vi "Convert State For Save.vi"(2 "Container State":T1, 3 "Display State":T2) -> (1 "Display State To Save":variant)   [LabVIEW 2017, in "XY Plot Matrix.xctl"]
uses:
  <vilib>/Math Plots/2D Math Plots/XY Plot Matrix/XY Plot Matrix XCtrl/XY Plot Matrix.xctl
  <vilib>/Math Plots/2D Math Plots/XY Plot Matrix/XY Plot Matrix XCtrl/State.ctl
  <vilib>/Math Plots/2D Math Plots/XY Plot Matrix/XY Plot Matrix/XY Plot Matrix.lvclass
  e:/builds/penguin/labview/branches/2017/dev/dist/vi.lib/Math Plots/2D Math Plots/2D Plot/2D Plot/2D Plot.lvclass
  <vilib>/Math Plots/2D Math Plots/2D Plot/Action String/XYPlotMatrix Ctrl Act Queue.ctl
  <vilib>/Math Plots/2D Math Plots/2D Plot/Action String/XYPlotMatrix Ctrl Act Cluster.ctl
  <vilib>/Math Plots/2D Math Plots/2D Plot/Action String/2DMathPlot State Class.ctl
  <vilib>/_xctls/Container State.ctl
  <vilib>/Math Plots/2D Math Plots/2D Plot/2D Plot/2D Plot.lvclass
  <vilib>/_xctls/XControlSupport.lvlib
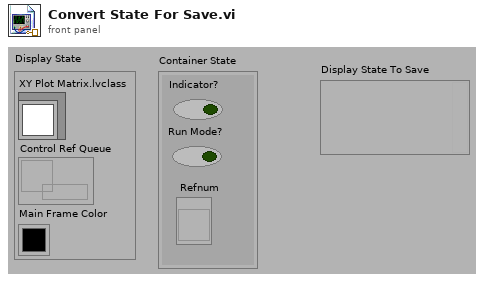
[diagram p1: front panel]
types:
  T1 = typedef "XControlSupport.lvlib/Container State.ctl" = cluster{"Indicator?":bool, "Run Mode?":bool, " Refnum":refnum<vi>}
  T2 = typedef "XY Plot Matrix.xctl/State.ctl" = cluster{"XY Plot Matrix.lvclass":refnum<class "XY Plot Matrix.lvclass">, "Control Ref Queue":T3, "Main Frame Color":u32}
  T3 = typedef "XYPlotMatrix Ctrl Act Queue.ctl" = refnum<queue>
  T4 = typedef "XYPlotMatrix Ctrl Act Cluster.ctl" = cluster{"Facade VI":refnum<vi>, "XControl":refnum<vi>, "Sub Panel":refnum<vi>, "Sub VI":refnum<vi>, "Export Image":refnum<vi>, "Display State Change Class":T5}
  T5 = typedef "2DMathPlot State Class.ctl" = enum16{"Update All (Undo)", "Update General", "Update Appearance", "Update Format", "Update Scale", "Update Marker", "Update Cursor", "None"}
  T6 = typedef "XY Plot Matrix.lvclass/Plotmatrix Property Array Cluster.ctl" = cluster{"Plotmatrix Property Array":T7, "Active Position":T11}
  T7 = typedef "XY Plot Matrix.lvclass/Plotmatrix Property Array.ctl" = T8[][]
  T8 = typedef "XY Plot Matrix.lvclass/Plotmatrix Property.ctl" = cluster{"Plot Property Array":T9}
  T9 = typedef "2D Plot.lvclass/Plot Property Array.ctl" = T10[]
  T10 = typedef "2D Plot.lvclass/Plot Property.ctl" = cluster{"Bar Plot Style":u8, "DigitalLineStyle":u8, "TransitionLocation":u8, "Transition Type":u8, "Fill To":i16, "Fill/Pt. Color":u32, "Label Style":u8, "Line Style":u8, "Line Width":u8, "Plot Color":u32, "Plot Interpolation":u8, "Plot Name":string, "Point Style":u8, "Visible?":bool, "XScaleIdx":u32, "YScaleIdx":u32}
  T11 = typedef "XY Plot Matrix.lvclass/Active Position.ctl" = cluster{"Row":i32, "Column":i32}
  T12 = typedef "2D Plot.lvclass/Property Cluster.ctl" = cluster{"Graph General":T13, "Format Property":string[], "Scale Array":T14, "Cursor Property":T17, "Annotation List":T19, "Active Cursor":i32, "Active Plot":i32}
  T13 = typedef "2D Plot.lvclass/Graph General Property.ctl" = cluster{"Palette Visible":cluster{"Graph Legend":bool, "Plot Legend":bool, "Auto size":bool, "Number of Plots":u32, "X Scrollbar":bool, "Scale Legend":bool, "Cursor Legend":bool}, "Plot Area Color":cluster{"FG Color":u32, "BG Color":u32}, "Bounds Size":cluster{"Width":u32, "Height":u32}, "Plot Area Bounds":cluster{"Left":i16, "Top":i16, "Right":i16, "Bottom":i16}}
  T14 = typedef "2D Plot.lvclass/Scale Array.ctl" = T15[]
  T15 = typedef "2D Plot.lvclass/Scale Cluster.ctl" = cluster{"General":cluster{"Editable":bool, "Flipped":bool, "Mapping Mode":u8, "Visible":bool, "Style":u8, "Scale Fit":u8}, "Offset and Multiplier":T16, "Range":cluster{"Minimum":dbl, "Maximum":dbl, "Increment":dbl, "Minor Increment":dbl, "Start":dbl}, "Tick Color":cluster{"Major Color":u32, "Minor Color":u32}, "Gird Color":cluster{"Major Color":u32, "Minor Color":u32}, "Marker":cluster{"Visible":bool, "FG Color":u32, "BG Color":u32, "Font Name":string, "Font Size":u32, "Font Bold":bool, "Font Italic":bool, "Font Strikeout":bool, "Font Underline":bool}, "Name Label":cluster{"Visible":bool, "FG Color":u32, "BG Color":u32, "Font Name":string, "Font Size":u32, "Font Bold":bool, "Font Italic":bool, "Font Strikeout":bool, "Font Underline":bool, "Justification":enum16{"Left", "Center", "Right"}, "Text":string}}
  T16 = typedef "LVOffsetAndMultiplierTypeDef.ctl" = cluster{"Offset":dbl, "Multiplier":dbl}
  T17 = typedef "2D Plot.lvclass/Cursor Property.ctl" = cluster{"Cursor List":T18, "Cursor List Addtional":cluster{"Cursor Selection Color":u32, "Line Style":u8, "Line Width":u8, "Visible":bool}[]}
  T18 = typedef "LVCursorListTypeDef.ctl" = cluster{"Name":string, "Color":u32, "Style":u8, "Point Style":u8, "Name Visible":bool, "Allow Drag":bool, "Cursor Mode":u32, "Plot":i32, "Index":i32, "Position":cluster{"X":dbl, "Y":dbl}, "X Scale":u32, "Y Scale":u32, "Watch Plots":i32[], "Watch All Plots":bool, "Plot Area":i32, "Label Offset":cluster{"X":dbl, "Y":dbl}}[]
  T19 = typedef "LVAnnotationListTypeDef.ctl" = cluster{"Name":string, "Color":u32, "Style":u8, "Point Style":u8, "Name Visible":bool, "Allow Drag":bool, "Annotation Mode":u32, "Plot":i32, "Index":i32, "Position":cluster{"X":dbl, "Y":dbl}, "X Scale":u32, "Y Scale":u32, "Show Arrow":bool, "Lock Name":bool, "Plot Area":i32, "Label Offset":cluster{"X":dbl, "Y":dbl}}[]
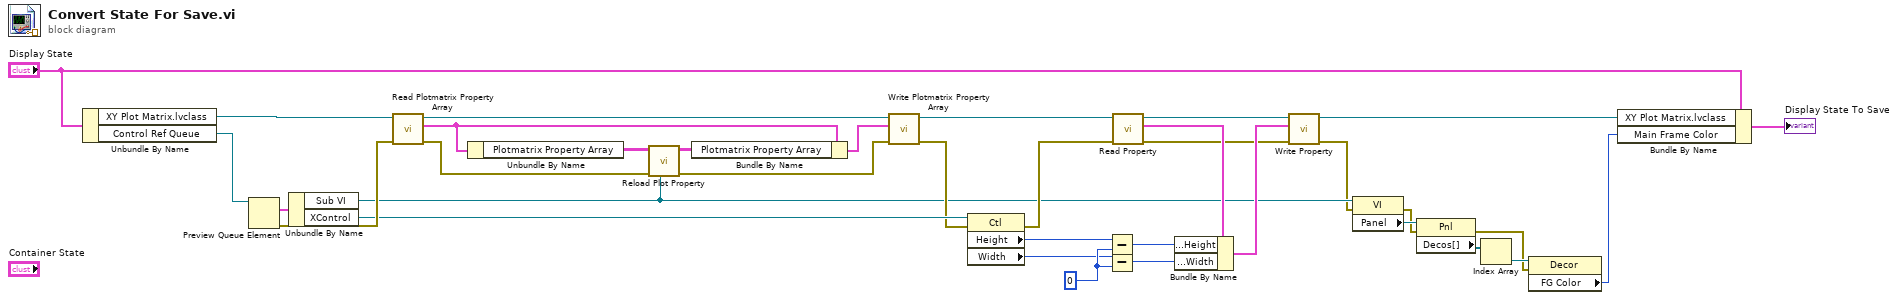
[diagram p0: block diagram]
diagram:
  w22 = u32 0 ("y")
  n1 = Unbundle By Name("Display State") -> ("XY Plot Matrix.lvclass"=w34:refnum<class "XY Plot Matrix.lvclass">, "Control Ref Queue"=w35:T3)
  n2 = Preview Queue Element(queue=w35) -> (element=w32:T4, error out=w29:errorcluster)  [unwired: 1 in, 3 out]
  n3 = Unbundle By Name(w32) -> ("Sub VI"=w8:refnum<vi>, "XControl"=w19:refnum<vi>)
  n4 = call <vilib>:"Read Plotmatrix Property Array.vi"("error in (no error)"=w29, "2D Plotmatrix.lvclass in"=w34) -> ("error out"=w28:errorcluster, "Plotmatrix Property Array Cluster"=w25:T6, "2D Plotmatrix.lvclass out"=w33:refnum<class "XY Plot Matrix.lvclass">)  [unwired: 7 out]
  n5 = Unbundle By Name(w25) -> ("Plotmatrix Property Array"=w26:T7)
  n6 = call <vilib>:"Reload Plot Property.vi"("Sub VI"=w8, "error in (no error)"=w28, "Plot Property Array In"=w26) -> ("error out"=w27:errorcluster, "Plot Property Array Out"=w24:T7)  [unwired: 7 out]
  n7 = Bundle By Name(cluster=w25, "Plotmatrix Property Array"=w24) -> (w23:T6)
  n8 = call <vilib>:"Write Plotmatrix Property Array.vi"("error in (no error)"=w27, "Plotmatrix Property Array Cluster"=w23, "2D Plotmatrix.lvclass in"=w33) -> ("error out"=w10:errorcluster, "2D Plotmatrix.lvclass out"=w18:refnum<class "XY Plot Matrix.lvclass">)  [unwired: 7 out]
  n9 = property class="Ctl"(reference=w19, error in=w10) -> (error out=w9:errorcluster, "Height"=w20:u32, "Width"=w21:u32)  [unwired: 1 out]
  n10 = Subtract(x=w20, y=w22) -> (x-y=w14:u32)
  n11 = Subtract(x=w21, y=w22) -> (x-y=w13:u32)
  n12 = call <vilib>:"Read Property.vi"("error in (no error)"=w9, "2D Plot.lvclass in"=w18) -> ("error out"=w11:errorcluster, "XY Graph Property Cluster"=w15:T12, "2D Plot.lvclass out"=w17:refnum<class "XY Plot Matrix.lvclass">)  [unwired: 7 out]
  n13 = Bundle By Name(cluster=w15, "Graph General.Bounds Size.Height"=w14, "Graph General.Bounds Size.Width"=w13) -> (w12:T12)
  n14 = call <vilib>:"Write Property.vi"("error in (no error)"=w11, "XY Graph Property Cluster"=w12, "2D Plot.lvclass in"=w17) -> ("error out"=w1:errorcluster, "2D Plot.lvclass out"=w16:refnum<class "XY Plot Matrix.lvclass">)  [unwired: 7 out]
  n15 = property class="VI"(reference=w8, error in=w1) -> (error out=w3:errorcluster, "Panel"=w7:refnum<vi>)  [unwired: 1 out]
  n16 = property class="Pnl"(reference=w7, error in=w3) -> (error out=w2:errorcluster, "Decos[]"=w6:refnum<vi>[])  [unwired: 1 out]
  n17 = Index Array(array=w6) -> (element=w5:refnum<vi>)  [unwired: 1 in]
  n18 = property class="Decor"(reference=w5, error in=w2) -> ("FG Color"=w4:u32)  [unwired: 2 out]
  n19 = Bundle By Name(cluster="Display State", "XY Plot Matrix.lvclass"=w16, "Main Frame Color"=w4) -> (→"Display State To Save":T2)
